vi "ble_read_message.vi"(8 "error in (no error)":errorcluster, 11 "COM Bluegiga in":refnum<visa-resource-name>) -> (0 "error out":errorcluster, 2 "message package":u8[](array[numeric]), 3 "COM Bluegiga out":refnum<visa-resource-name>)   [LabVIEW 2017]
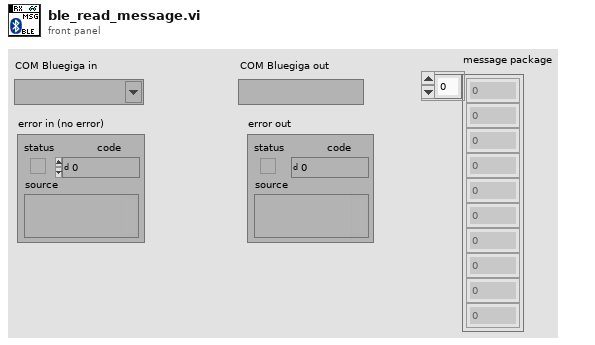
[diagram p1: front panel]
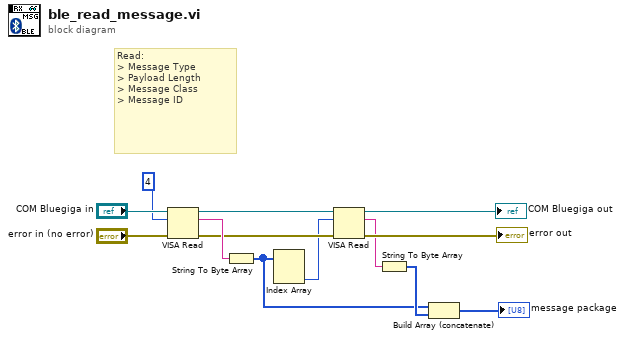
[diagram p0: block diagram]
diagram:
  # "Read:\n> Message Type\n> Payload Length\n> Message Class\n> Message ID"
  n1 = VISA Read(VISA resource name="COM Bluegiga in", byte count=u32 4, error in (no error)="error in (no error)") -> (VISA resource name out=w8:refnum<visa-resource-name>, read buffer=w10:string, error out=w9:errorcluster)  [unwired: 1 out]
  n2 = String To Byte Array(string=w10) -> (unsigned byte array=w1:u8[])
  n3 = Index Array(array=w1) -> (element #2=w5:u8)  [unwired: 2 in, 1 out]
  n4 = VISA Read(VISA resource name=w8, byte count=w5, error in (no error)=w9) -> (VISA resource name out=→"COM Bluegiga out":refnum<visa-resource-name>, read buffer=w4:string, error out=→"error out":errorcluster)  [unwired: 1 out]
  n5 = String To Byte Array(string=w4) -> (unsigned byte array=w2:u8[])
  n6 = Build Array (concatenate)(w1, w2) -> (→"message package":u8[])
